vi "Recepción_Producto_Dídier Javier Ramírez Henao.vi"() -> ()   [LabVIEW 2020]
panel:
  out "PARADA 1":bool
  out "FIN":bool
  out "DESCARGUE":bool
  out "ALMACENA":bool
  out "SUMINISTRO":bool
  out "RECEPCIÓN":bool
  out "INICIO":bool
  in  "Cancel 2":bool
  in  "stop":bool
  out "Silo 2":dbl(slide) scale=0.0..50.0
  out "Silo 1":dbl(slide) scale=0.0..50.0
  out "B4":bool
  out "B3":bool
  out "B2":bool
  out "B1":bool
  in  "Marcha 1":bool
  # "Dídier Javier Ramírez Henao"
  # "Subproceso 1: Recepción del producto"
  # "Almacenamiento"
  # "Almacenamiento"
  # "Zona de recepción del producto en grano"
  # "Banda transportadora 1"
  # "Banda transportadora 2"
  # "Banda transportadora 3"
  # "Banda transportadora 4"
  # "Bandas de descargue del producto"
  # "Pulsadores de mando"
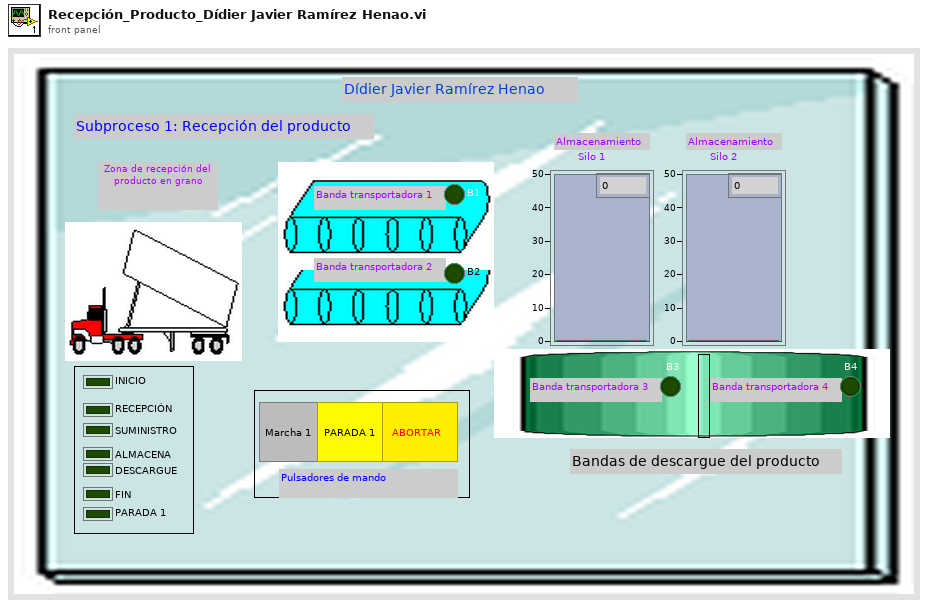
[diagram p1: front panel]
types:
  T1 = enum16{"INICIO", "RECEPCIÓN", "SUMINISTRO", "ALMACENAMIENTO", "DESCARGUE", "FIN", "PAUSA"}
  T2 = enum16{"INICIO", "RECEPCIÓN", "SUMINISTRO", "ALMACENAMIENTO", "DESCARGUE", "FIN"}
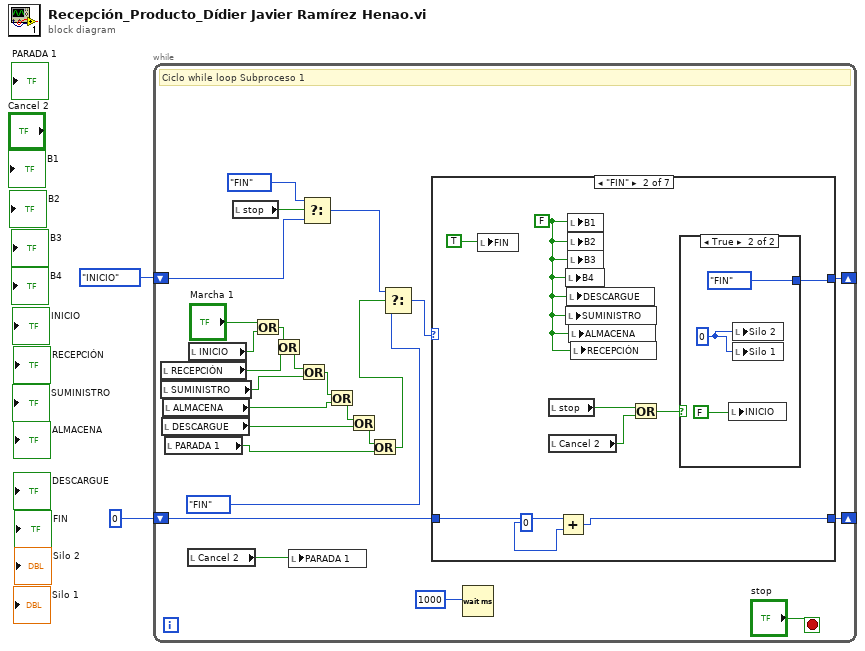
[diagram p0: block diagram]
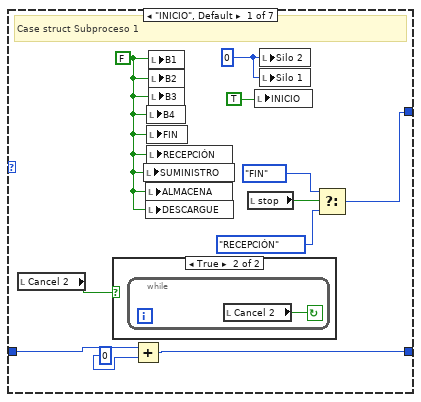
[diagram p2: hidden frame]
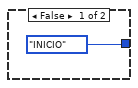
[diagram p4: hidden frame]
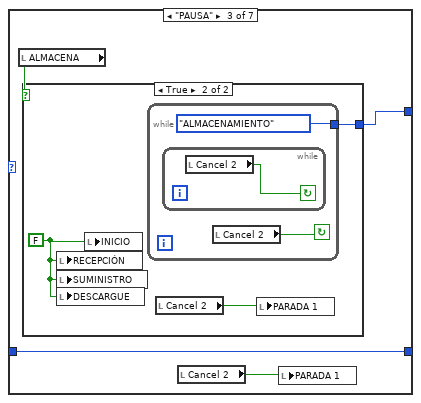
[diagram p5: hidden frame]
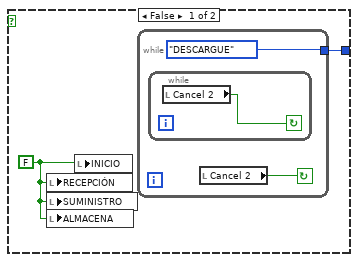
[diagram p6: hidden frame]
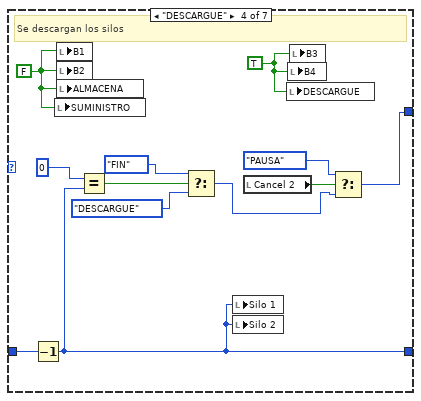
[diagram p7: hidden frame]
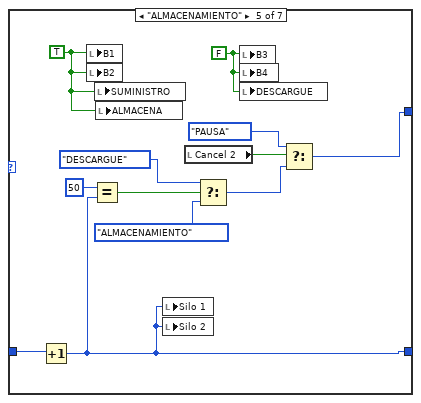
[diagram p8: hidden frame]
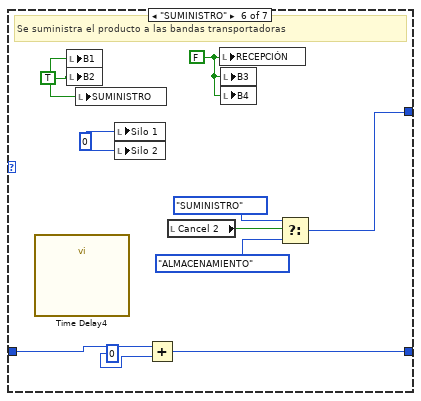
[diagram p9: hidden frame]
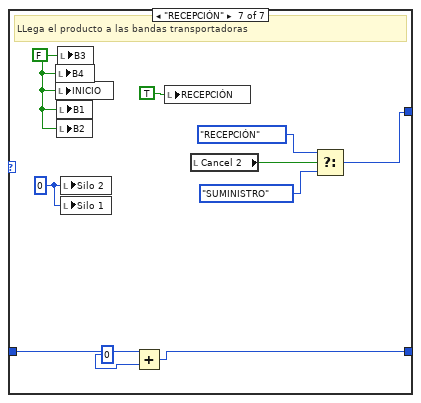
[diagram p10: hidden frame]
diagram:
  n1 = while {
    shift-right: [w27] -> _
    shift-left: T1."INICIO" -> [w5]
    shift-right: [w23] -> _
    shift-left: 0 -> [w24]
    stop <- "stop" stop-if-true
    # "Ciclo while loop Subproceso 1"
    n2 = local read "RECEPCIÓN"() -> (w18:bool)
    n3 = local read "SUMINISTRO"() -> (w16:bool)
    n4 = local read "DESCARGUE"() -> (w12:bool)
    n5 = local read "ALMACENA"() -> (w14:bool)
    n6 = local read "PARADA 1"() -> (w9:bool)
    n7 = local read "Cancel 2"() -> (w3:bool)
    n8 = local read "INICIO"() -> (w20:bool)
    n9 = local read "stop"() -> (w6:bool)
    n10 = Or(x="Marcha 1", y=w20) -> (x .or. y?=w19:bool)
    n11 = Or(x=w19, y=w18) -> (x .or. y?=w17:bool)
    n12 = local write "PARADA 1"(w3) -> ()
    n13 = Or(x=w17, y=w16) -> (x .or. y?=w15:bool)
    n14 = Select(t=T1."FIN", s=w6, f=w5) -> (s? t:f=w4:T1)
    n15 = Or(x=w15, y=w14) -> (x .or. y?=w13:bool)
    n16 = Or(x=w13, y=w12) -> (x .or. y?=w10:bool)
    n17 = Or(x=w10, y=w9) -> (x .or. y?=w8:bool)
    n18 = Select(t=w4, s=w8, f=T2."FIN") -> (s? t:f=w22:T1)
    n19 = case shown="\"FIN\"" w22 {
      tunnel: [w30 w44 w55 w71 w84 w101 w106] -> w27
      tunnel: w24 -> [w36 w48 w56 w79 w88 w97 w110]
      tunnel: [w37 w46 w56 w77 w87 w96 w108] -> w23
      frame "INICIO", Default {
        w38 = 0
        w33 = FALSE
        # "Case struct Subproceso 1"
        n20 = local read "Cancel 2"() -> (w28:bool)
        n21 = case shown="True" w28 {
          frame False {
          }
          frame True {
            n22 = while {
              stop <- w39 continue-if-true
              n23 = local read "Cancel 2"() -> (w39:bool)
            }
          }
        }
        n24 = Add(x=w36, y=0) -> (x+y=w37:i32)
        n25 = local write "SUMINISTRO"(w33) -> ()
        n26 = local write "ALMACENA"(w33) -> ()
        n27 = local write "DESCARGUE"(w33) -> ()
        n28 = local write "B4"(w33) -> ()
        n29 = local write "FIN"(w33) -> ()
        n30 = local write "RECEPCIÓN"(w33) -> ()
        n31 = local write "B1"(w33) -> ()
        n32 = local write "B2"(w33) -> ()
        n33 = local write "B3"(w33) -> ()
        n34 = local read "stop"() -> (w32:bool)
        n35 = local write "INICIO"(TRUE) -> ()
        n36 = local write "Silo 2"(w38) -> ()
        n37 = local write "Silo 1"(w38) -> ()
        n38 = Select(t=T1."FIN", s=w32, f=T1."RECEPCIÓN") -> (s? t:f=w30:T1)
      }
      frame "FIN" {
        w43 = FALSE
        n39 = local write "FIN"(TRUE) -> ()
        n40 = local read "stop"() -> (w41:bool)
        n41 = local read "Cancel 2"() -> (w40:bool)
        n42 = Add(x=w48, y=0) -> (x+y=w46:i32)
        n43 = local write "B4"(w43) -> ()
        n44 = local write "SUMINISTRO"(w43) -> ()
        n45 = local write "DESCARGUE"(w43) -> ()
        n46 = local write "B1"(w43) -> ()
        n47 = local write "B2"(w43) -> ()
        n48 = local write "B3"(w43) -> ()
        n49 = local write "ALMACENA"(w43) -> ()
        n50 = local write "RECEPCIÓN"(w43) -> ()
        n51 = Or(x=w41, y=w40) -> (x .or. y?=w42:bool)
        n52 = case shown="True" w42 {
          tunnel: [T1."INICIO" T1."FIN"] -> w44
          frame False {
          }
          frame True {
            w50 = 0
            n53 = local write "INICIO"(FALSE) -> ()
            n54 = local write "Silo 2"(w50) -> ()
            n55 = local write "Silo 1"(w50) -> ()
          }
        }
      }
      frame "PAUSA" {
        n56 = local read "ALMACENA"() -> (w54:bool)
        n57 = case shown="True" w54 {
          tunnel: [w58 w64] -> w55
          frame False {
            w57 = FALSE
            n58 = local write "RECEPCIÓN"(w57) -> ()
            n59 = local write "SUMINISTRO"(w57) -> ()
            n60 = local write "ALMACENA"(w57) -> ()
            n61 = local write "INICIO"(w57) -> ()
            n62 = while {
              tunnel: [T1."DESCARGUE"] -> w58
              stop <- w59 continue-if-true
              n63 = while {
                stop <- w61 continue-if-true
                n64 = local read "Cancel 2"() -> (w61:bool)
              }
              n65 = local read "Cancel 2"() -> (w59:bool)
            }
          }
          frame True {
            w63 = FALSE
            n66 = local write "RECEPCIÓN"(w63) -> ()
            n67 = local write "SUMINISTRO"(w63) -> ()
            n68 = local write "DESCARGUE"(w63) -> ()
            n69 = local write "INICIO"(w63) -> ()
            n70 = while {
              tunnel: [T1."ALMACENAMIENTO"] -> w64
              stop <- w65 continue-if-true
              n71 = while {
                stop <- w67 continue-if-true
                n72 = local read "Cancel 2"() -> (w67:bool)
              }
              n73 = local read "Cancel 2"() -> (w65:bool)
            }
            n74 = local read "Cancel 2"() -> (w62:bool)
            n75 = local write "PARADA 1"(w62) -> ()
          }
        }
        n76 = local read "Cancel 2"() -> (w53:bool)
        n77 = local write "PARADA 1"(w53) -> ()
      }
      frame "DESCARGUE" {
        w76 = TRUE
        w75 = FALSE
        # "Se descargan los silos"
        n78 = Decrement(x=w79) -> (x-1=w77:i32)
        n79 = local write "SUMINISTRO"(w75) -> ()
        n80 = local write "B1"(w75) -> ()
        n81 = local write "B2"(w75) -> ()
        n82 = local write "ALMACENA"(w75) -> ()
        n83 = Equal?(x=0, y=w77) -> (x = y?=w74:bool)
        n84 = Select(t=T1."FIN", s=w74, f=T1."DESCARGUE") -> (s? t:f=w72:T1)
        n85 = local write "Silo 1"(w77) -> ()
        n86 = local write "Silo 2"(w77) -> ()
        n87 = local read "Cancel 2"() -> (w73:bool)
        n88 = local write "DESCARGUE"(w76) -> ()
        n89 = local write "B4"(w76) -> ()
        n90 = local write "B3"(w76) -> ()
        n91 = Select(t=T1."PAUSA", s=w73, f=w72) -> (s? t:f=w71:T1)
      }
      frame "ALMACENAMIENTO" {
        w80 = FALSE
        w91 = TRUE
        n92 = Increment(x=w88) -> (x+1=w87:i32)
        n93 = local write "B1"(w91) -> ()
        n94 = local write "B2"(w91) -> ()
        n95 = Equal?(x=50, y=w87) -> (x = y?=w90:bool)
        n96 = local write "SUMINISTRO"(w91) -> ()
        n97 = local write "ALMACENA"(w91) -> ()
        n98 = local write "Silo 1"(w87) -> ()
        n99 = local write "Silo 2"(w87) -> ()
        n100 = local read "Cancel 2"() -> (w86:bool)
        n101 = Select(t=T1."DESCARGUE", s=w90, f=T1."ALMACENAMIENTO") -> (s? t:f=w85:T1)
        n102 = local write "B3"(w80) -> ()
        n103 = local write "B4"(w80) -> ()
        n104 = local write "DESCARGUE"(w80) -> ()
        n105 = Select(t=T1."PAUSA", s=w86, f=w85) -> (s? t:f=w84:T1)
      }
      frame "SUMINISTRO" {
        w94 = 0
        w99 = FALSE
        w100 = TRUE
        # "Se suministra el producto a las bandas transportadoras"
        n106 = call "Time Delay4"() -> ()  [unwired: 11 in, 1 out]
        n107 = local write "B1"(w100) -> ()
        n108 = local write "B2"(w100) -> ()
        n109 = local write "SUMINISTRO"(w100) -> ()
        n110 = local write "Silo 1"(w94) -> ()
        n111 = local write "Silo 2"(w94) -> ()
        n112 = Add(x=w97, y=0) -> (x+y=w96:i32)
        n113 = local read "Cancel 2"() -> (w98:bool)
        n114 = local write "RECEPCIÓN"(w99) -> ()
        n115 = local write "B3"(w99) -> ()
        n116 = local write "B4"(w99) -> ()
        n117 = Select(t=T1."SUMINISTRO", s=w98, f=T1."ALMACENAMIENTO") -> (s? t:f=w101:T1)
      }
      frame "RECEPCIÓN" {
        w111 = 0
        w105 = FALSE
        # "LLega el producto a las bandas transportadoras"
        n118 = local write "B4"(w105) -> ()
        n119 = local write "INICIO"(w105) -> ()
        n120 = local write "B1"(w105) -> ()
        n121 = local write "B2"(w105) -> ()
        n122 = local write "B3"(w105) -> ()
        n123 = local write "Silo 2"(w111) -> ()
        n124 = local write "Silo 1"(w111) -> ()
        n125 = Add(x=w110, y=0) -> (x+y=w108:i32)
        n126 = local write "RECEPCIÓN"(TRUE) -> ()
        n127 = local read "Cancel 2"() -> (w107:bool)
        n128 = Select(t=T1."RECEPCIÓN", s=w107, f=T1."SUMINISTRO") -> (s? t:f=w106:T1)
      }
    }
    n129 = Wait (ms)(milliseconds to wait=1000) -> ()  [unwired: 1 out]
  }
